vi "TDT-Read Tag.vi"(0 "RPcox":refnum<k7>, 5 "Name":string, 11 "error in":errorcluster) -> (4 "RPcox Out":refnum<k7>, 8 "GetTagVal":sgl, 15 "error out":errorcluster)   [LabVIEW 2020]
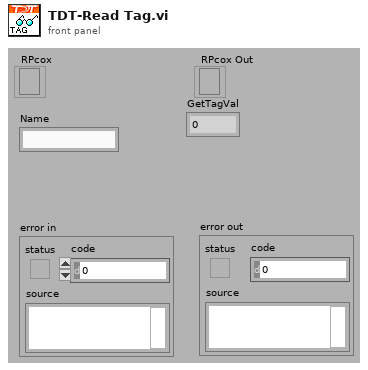
[diagram p1: front panel]
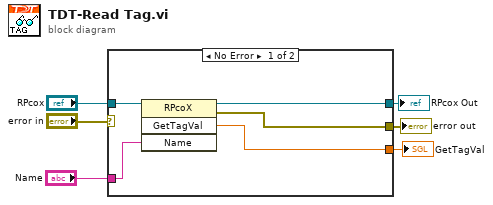
[diagram p0: block diagram]
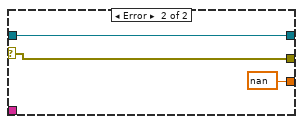
[diagram p2: hidden frame]
diagram:
  n1 = case shown="No Error" "error in" {
    selector: "error in" -> [_ w14]
    tunnel: "RPcox" -> [w10 w13]
    tunnel: [w9 w14] -> w5
    tunnel: [w11 w13] -> w4
    tunnel: "Name" -> [w8 _]
    tunnel: [w7 sgl nan] -> w1
    frame No Error {
      n2 = invoke class="RPcoX" method="GetTagVal"(reference=w10, "Name"=w8) -> (reference out=w11:refnum<k7>, error out=w9:errorcluster, "GetTagVal"=w7:sgl)  [unwired: 2 in, 1 out]
    }
    frame Error {
    }
  }
  "error out" <- w5
  "RPcox Out" <- w4
  "GetTagVal" <- w1
